vi "Get Gyro Angle.vi"(11 "GyroDevRef":T1={"DevStatus"={"status"=FALSE, "code"=0, "source"=""}, "Analog Module"=enum."Controller 1", "Analog Channel"=enum."AI 1", "Offset"=0.0, "Gain (VoltsPerDegree/Second)"=0.0}) -> (0 "Angular Rate":dbl, 1 "Angle":dbl, 3 "GyroDevRef 2":T1={"DevStatus"={"status"=FALSE, "code"=0, "source"=""}, "Analog Module"=enum."Controller 1", "Analog Channel"=enum."AI 1", "Offset"=0.0, "Gain (VoltsPerDegree/Second)"=0.0})   [LabVIEW 2014]
uses:
  <vilib>/Rock Robotics/WPI/Gyro/WPI_GyroDevRef.ctl
  <vilib>/Rock Robotics/SystemInterfaces/Typedef/FPGA_TypedefAnalogModule.ctl
  <vilib>/Rock Robotics/SystemInterfaces/AI/FPGA_AIChannel.ctl
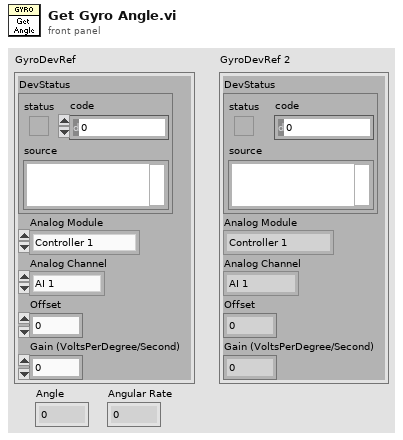
[diagram p1: front panel]
types:
  T1 = typedef "WPI_GyroDevRef.ctl" = cluster{"DevStatus":errorcluster, "Analog Module":T2, "Analog Channel":T3, "Offset":dbl, "Gain (VoltsPerDegree/Second)":dbl}
  T2 = typedef "FPGA_TypedefAnalogModule.ctl" = enum16{"Controller 1"}
  T3 = typedef "FPGA_AIChannel.ctl" = enum8{"AI 0", "AI 1", "AI 2", "AI 3", "AI MXP 0", "AI MXP 1", "AI MXP 2", "AI MXP 3", "Invalid"}
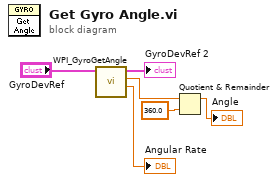
[diagram p0: block diagram]
diagram:
  n1 = call <vilib>:"WPI_GyroGetAngle.vi"("GyroDevRef"="GyroDevRef") -> ("Angular Rate"=→"Angular Rate":dbl, "Angle"=w6:dbl, "GyroDevRef"=→"GyroDevRef 2":T1)  [unwired: 7 in, 1 out]
  n2 = Quotient & Remainder(x=w6, y=360.0) -> (x-y*floor(x/y)=→"Angle":dbl)  [unwired: 1 out]
